vi "_SetBitfiledValue.vi"(7 "bitfield value":variant, 8 "error in (no error)":errorcluster, 9 "size":i32, 10 "offset":i32, 11 "soft value":u64) -> (0 "error out":errorcluster, 2 "mask":u64 format="%.0x", 3 "update value":u64)   [LabVIEW 2015, in "Bitfield.lvlib"]
uses:
  Bitfield.lvlib
  <vilib>/Utility/Data Type/NI_Data Type.lvlib
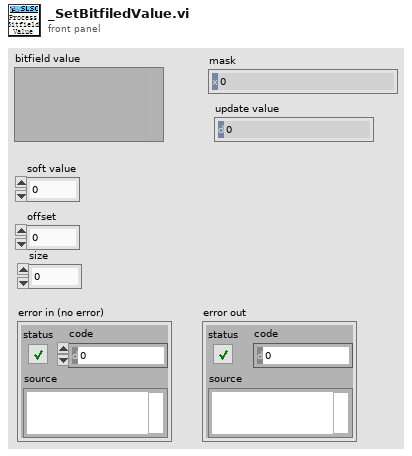
[diagram p1: front panel]
types:
  T1 = typedef "NI_Data Type.lvlib/Data Type.ctl" = enum8{"Invalid Type", "Void", "I8", "I16", "I32", "I64", "U8", "U16", "U32", "U64", "Single Float", "Double Float", "Extended Float", "Single Complex", "Double Complex", "Extended Complex", "Enum U8", "Enum U16", "Enum U32", "Enum U64", "Single Float With Unit", "Double Float With Unit", "Extended Float With Unit", "Single Complex with Unit", "Double Complex with Unit", "Extended Complex with Unit", "Boolean", "String", "Path", "Picture", "Tag", "Array", "Cluster", "Variant", "LV Variant", "Waveform", "Timestamp", "Digital Waveform", "Digital Data", "ExpressData", "Refnum", "External Data", "VI", "Poly VI", "LabVIEW Class Instance", "Fixed Point"}
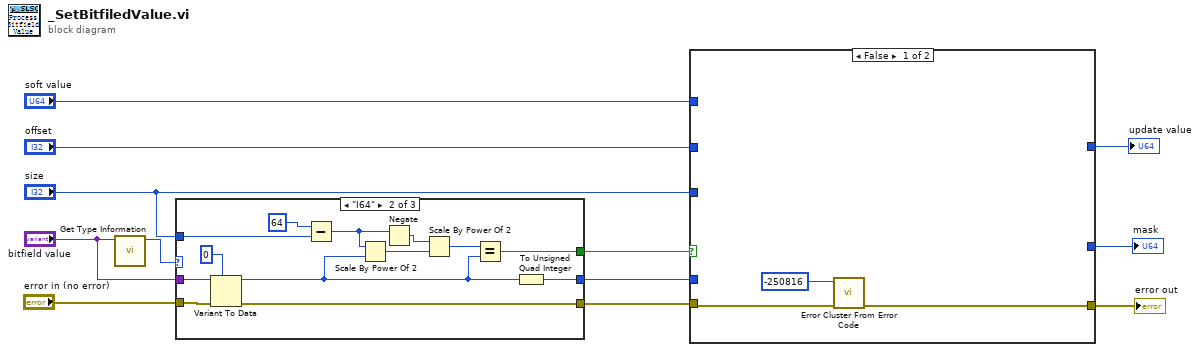
[diagram p0: block diagram]
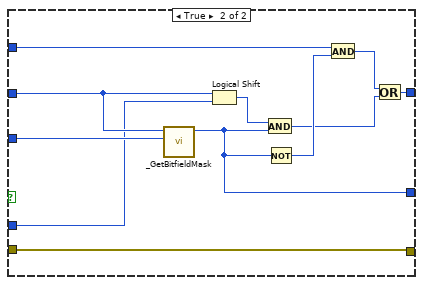
[diagram p2: hidden frame]
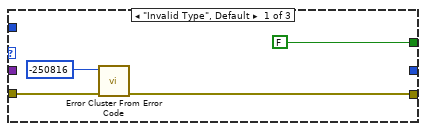
[diagram p3: hidden frame]
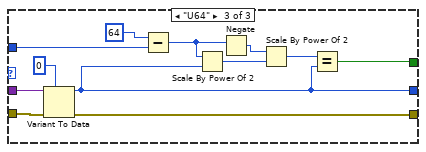
[diagram p4: hidden frame]
diagram:
  n1 = call <vilib>:"Get Type Information.vi"("Variant"="bitfield value") -> ("Type"=w9:T1)  [unwired: 6 in, 4 out]
  n2 = case shown="\"I64\"" w9 {
    tunnel: "bitfield value" -> [_ w29 w41]
    tunnel: "error in (no error)" -> [w15 w28 w40]
    tunnel: [_ w25 w30] -> w5
    tunnel: [w14 w26 w38] -> w2
    tunnel: "size" -> [_ w19 w32]
    tunnel: [FALSE w17 w31] -> w3
    frame "Invalid Type", Default {
      n3 = call <vilib>:"Error Cluster From Error Code.vi"("error in (no error)"=w15, "error code (0)"=-250816) -> ("error out"=w14:errorcluster)  [unwired: 7 in]
    }
    frame "I64" {
      n4 = Variant To Data(error in=w28, type=i64 0, Variant=w29) -> (data=w18:i64, error out=w26:errorcluster)
      n5 = Subtract(x=64, y=w19) -> (x-y=w21:i32)
      n6 = Scale By Power Of 2(n=w21, x=w18) -> (x*2^n=w23:i64)
      n7 = Negate(x=w21) -> (-x=w24:i32)
      n8 = Scale By Power Of 2(n=w24, x=w23) -> (x*2^n=w20:i64)
      n9 = Equal?(x=w20, y=w18) -> (x = y?=w17:bool)
      n10 = To Unsigned Quad Integer(1:w18) -> (0:w25:u64)
    }
    frame "U64" {
      n11 = Variant To Data(error in=w40, type=u64 0, Variant=w41) -> (data=w30:u64, error out=w38:errorcluster)
      n12 = Subtract(x=64, y=w32) -> (x-y=w34:i32)
      n13 = Scale By Power Of 2(n=w34, x=w30) -> (x*2^n=w36:u64)
      n14 = Negate(x=w34) -> (-x=w37:i32)
      n15 = Scale By Power Of 2(n=w37, x=w36) -> (x*2^n=w33:u64)
      n16 = Equal?(x=w33, y=w30) -> (x = y?=w31:bool)
    }
  }
  n17 = case shown="False" w3 {
    tunnel: [_ w55] -> w12
    tunnel: "soft value" -> [_ w54]
    tunnel: [_ w53] -> w10
    tunnel: "offset" -> [_ w48]
    tunnel: "size" -> [_ w47]
    tunnel: w5 -> [_ w46]
    tunnel: w2 -> [w43 w45]
    tunnel: [w42 w45] -> w1
    frame False {
      n18 = call <vilib>:"Error Cluster From Error Code.vi"("error in (no error)"=w43, "error code (0)"=-250816) -> ("error out"=w42:errorcluster)  [unwired: 7 in]
    }
    frame True {
      n19 = call "_GetBitfieldMask.vi"("size"=w47, "offset"=w48) -> ("mask"=w53:u64)  [unwired: 9 in]
      n20 = Logical Shift(y=w48, x=w46) -> (x << y=w51:u64)
      n21 = And(x=w51, y=w53) -> (x .and. y?=w49:u64)
      n22 = Not(x=w53) -> (.not. x?=w52:u64)
      n23 = And(x=w54, y=w52) -> (x .and. y?=w50:u64)
      n24 = Or(x=w50, y=w49) -> (x .or. y?=w55:u64)
    }
  }
  "update value" <- w12
  "error out" <- w1
  "mask" <- w10
